vi "SET Message.vi"(8 "error in (no error)":errorcluster, 10 "Data":string, 11 "Child_2_Class in":refnum<class "Console_Class.lvclass">) -> (0 "error out":errorcluster, 3 "Child_2_Class out":refnum<class "Console_Class.lvclass">)   [LabVIEW 2023, in "Console_Actor.lvlib" / "Console_Class.lvclass"]
uses:
  Console_Class.lvclass
  Usr Ev/Child_2 - Ctrl - Enum - Events (Temp).ctl
  Console_Class.lvclass/Console_Class.ctl
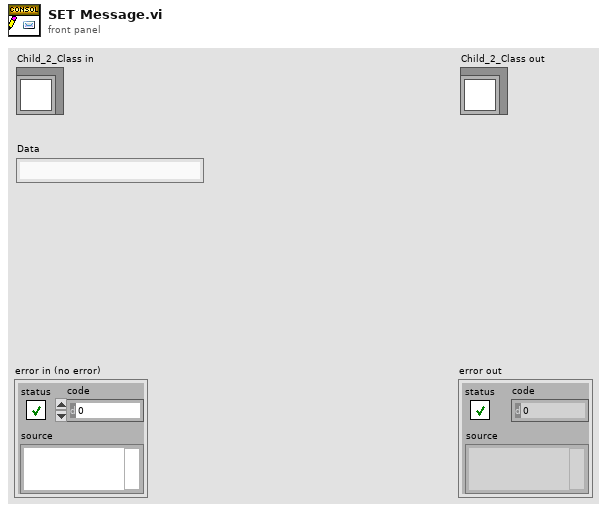
[diagram p1: front panel]
types:
  T1 = typedef "Console_Actor.lvlib/Console_Class.lvclass/Child_2 - Ctrl - Enum - Events (Temp).ctl" = enum16{"SEND MESSAGE Ev", "STOP_ACTOR Ev", "INIT_ACTOR Ev", "START Ev", "STOP Ev", "GET Ev", "SET Ev", "ERROR_HANDLER Ev", "RESET Ev", "T2 Ev", "T3 Ev", "T4 Ev"}
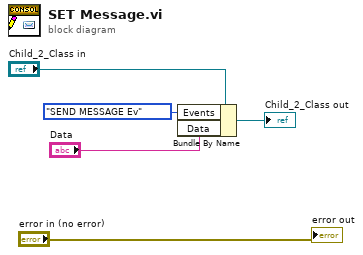
[diagram p0: block diagram]
diagram:
  n1 = Bundle By Name(cluster="Child_2_Class in", "Events"=Child_2_-_Ctrl_-_Enum_-_Events_(Temp)."SEND MESSAGE Ev" ("Child Trigger Event Cluster.Events"), "Data"="Data") -> (→"Child_2_Class out":refnum<class "Console_Class.lvclass">)
  "error out" <- "error in (no error)"
